vi "Append Text Table to Report.vi"(0 "report in":refnum<class "NI_Standard Report.lvclass">, 1 "column width (1)":dbl=1.0 format="%.2f", 2 "measurement system":u16(ring)=2 caption="measurement system for column width (Default)" items=["US", "Metric", "Default"], 3 "MS Office parameters":T2, 5 "column headers":string[](array[string]), 7 "row headers":string[](array[string]), 9 "text data":string[][](array[string]), 11 "error in (no error)":errorcluster, 13 "separate page?":bool, 14 "show grid lines":bool=TRUE) -> (4 "report out":refnum<class "NI_Standard Report.lvclass">, 8 "range (wd) - start (xl)":T1, 10 "end (xl)":cluster{"row (xl) ":i32, "col (xl) ":i32}, 15 "error out":errorcluster)   [LabVIEW 2017, in "NI_Standard Report.lvclass"]
doc: "Appends a 2D array to a report as a table with the given column width. You can use this polymorphic VI to append an array of strings or numbers. The data type you wire to the <B>text data</B> input determines the polymorphic instance to use."
uses:
  <vilib>/Utility/NIReport.llb/Standard Report/NI_Standard Report.lvclass
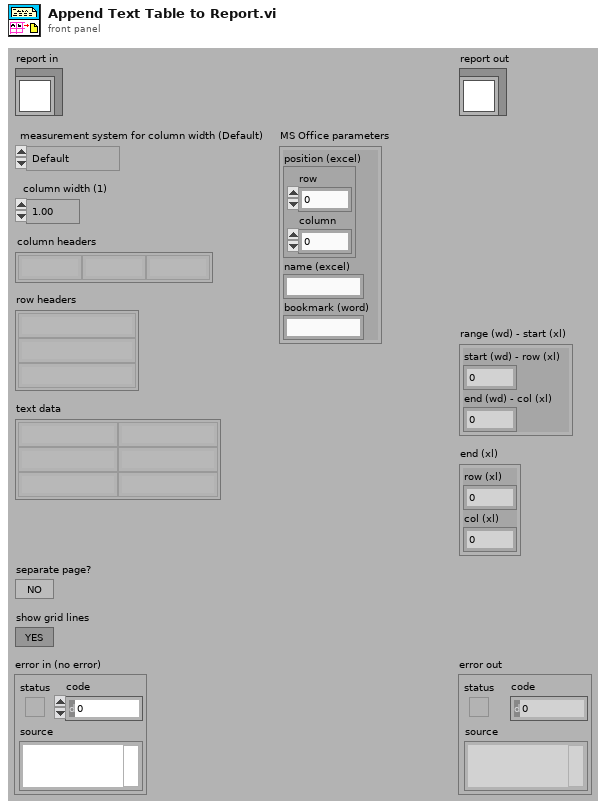
[diagram p1: front panel]
types:
  T1 = cluster{"start (wd) - row (xl) ":i32, "end (wd) - col (xl) ":i32}
  T2 = cluster{"position (excel)":cluster{"row":i32, "column":i32}, "name (excel)":string, "bookmark (word)":string}
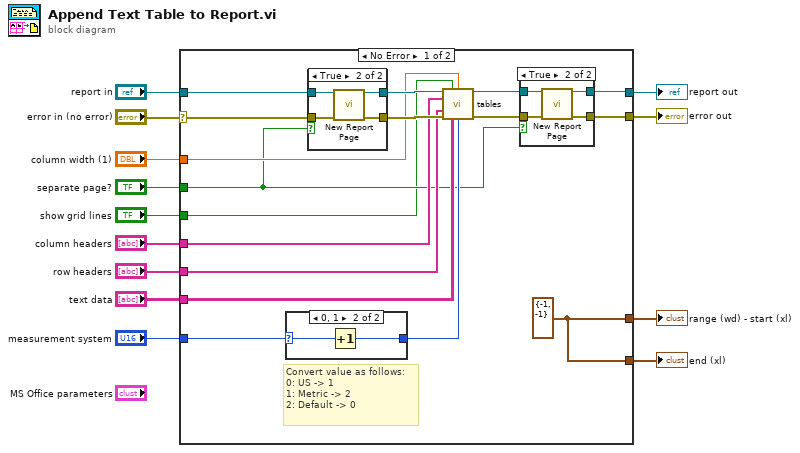
[diagram p0: block diagram]
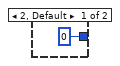
[diagram p2: hidden frame]
diagram:
  n1 = case shown="No Error" "error in (no error)" {
    selector: "error in (no error)" -> [w23 w47]
    tunnel: [w22 w47] -> w12
    tunnel: [w24 w46] -> w10
    tunnel: "report in" -> [w25 w46]
    tunnel: [w21 _] -> w9
    tunnel: [w21 _] -> w8
    tunnel: "column width (1)" -> [w20 _]
    tunnel: "measurement system" -> [w19 _]
    tunnel: "text data" -> [w18 _]
    tunnel: "column headers" -> [w17 _]
    tunnel: "row headers" -> [w16 _]
    tunnel: "separate page?" -> [w15 _]
    tunnel: "show grid lines" -> [w14 _]
    frame No Error {
      w21 = cluster{"row (xl)":i32, "col (xl)":i32} {"row (xl)"=-1, "col (xl)"=-1} ("end (xl)")
      # "Convert value as follows:\n0: US -> 1\n1: Metric -> 2\n2: Default -> 0"
      n2 = case shown="0, 1" w19 {
        selector: w19 -> [_ w33]
        tunnel: [u16 0 w32] -> w30
        frame 2, Default {
        }
        frame 0, 1 {
          n3 = Increment(x=w33) -> (x+1=w32:u16)
        }
      }
      n4 = case shown="True" w15 {
        tunnel: w25 -> [w41 w45]
        tunnel: w23 -> [w40 w44]
        tunnel: [w41 w43] -> w26
        tunnel: [w40 w42] -> w27
        frame False {
        }
        frame True {
          n5 = call-dynamic "New Report Page.vi"("report in"=w45, "error in (no error)"=w44) -> ("report out"=w43:refnum<class "NI_Standard Report.lvclass">, "error out"=w42:errorcluster)  [unwired: 1 in, 11 out]
        }
      }
      n6 = call <vilib>:"tables.vi"("report in"=w26, "show grid lines"=w14, "column width"=w20, "column headers"=w17, "row headers"=w16, "error in (no error)"=w27, "text data"=w18, "Measurement System"=w30) -> ("report out"=w29:refnum<class "NI_Standard Report.lvclass">, "error out"=w28:errorcluster)  [unwired: 6 out]
      n7 = case shown="True" w15 {
        tunnel: w29 -> [w35 w39]
        tunnel: w28 -> [w34 w38]
        tunnel: [w35 w37] -> w24
        tunnel: [w34 w36] -> w22
        frame False {
        }
        frame True {
          n8 = call-dynamic "New Report Page.vi"("report in"=w39, "error in (no error)"=w38) -> ("report out"=w37:refnum<class "NI_Standard Report.lvclass">, "error out"=w36:errorcluster)  [unwired: 1 in, 11 out]
        }
      }
    }
    frame Error {
    }
  }
  "error out" <- w12
  "report out" <- w10
  "end (xl)" <- w8
  "range (wd) - start (xl)" <- w9
